vi "Write Prompt Stop.vi"(8 "error in (no error)":errorcluster, 10 "Stop Button":bool, 11 "Generic Instrument in":refnum<class "Generic Instrument.lvclass">) -> (0 "error out":errorcluster, 3 "Generic Instrument out":refnum<class "Generic Instrument.lvclass">)   [LabVIEW 2014, in "Generic Instrument.lvlib" / "Generic Instrument.lvclass"]
uses:
  Generic Instrument.lvclass
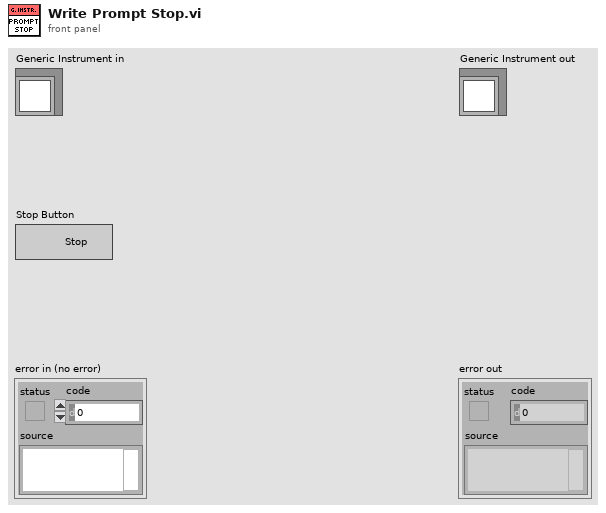
[diagram p1: front panel]
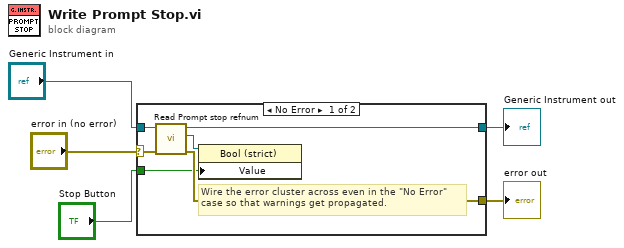
[diagram p0: block diagram]
diagram:
  n1 = case shown="No Error" "error in (no error)" {
    selector: "error in (no error)" -> [w9 w13]
    tunnel: [w8 w13] -> w4
    tunnel: [w10 w12] -> w2
    tunnel: "Generic Instrument in" -> [w11 w12]
    tunnel: "Stop Button" -> [w6 _]
    frame No Error {
      # "Wire the error cluster across even in the \"No Error\"\ncase so that warnings get propagated."
      n2 = call-dynamic "Read Prompt stop refnum.vi"("error in (no error)"=w9, "Generic Instrument in"=w11) -> ("error out"=w8:errorcluster, "Prompt stop refnum"=w7:refnum<vi>, "Generic Instrument out"=w10:refnum<class "Generic Instrument.lvclass">)  [unwired: 7 in]
      n3 = property class="Bool (strict)"(reference=w7, "Value"=w6) -> ()  [unwired: 1 in, 2 out]
    }
    frame Error {
    }
  }
  "error out" <- w4
  "Generic Instrument out" <- w2
